vi "Parse Hexadecimal String.vi"(11 "Hex String":string) -> (3 "Bit Stream":bool[](array[boolean]))   [LabVIEW 2019, in "Day 16.lvlib"]
uses:
  Day 16.lvlib
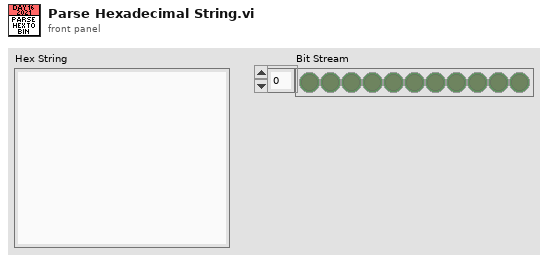
[diagram p1: front panel]
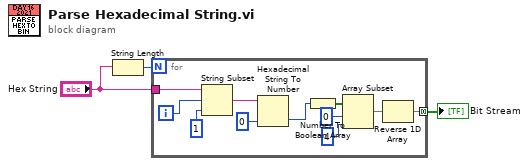
[diagram p0: block diagram]
diagram:
  n1 = String Length(string="Hex String") -> (length=w1:i32)
  n2 = for {
    N: w1 -> [_]
    tunnel: "Hex String" -> [w14]
    tunnel: [w4] -> w3 mode=concatenating
    i -> [w12]
    n3 = String Subset(string=w14, offset (0)=w12, length (rest)=1 ("length (rest)")) -> (substring=w11:string)
    n4 = Hexadecimal String To Number(string=w11, default (0uL)=u8 0 ("default (0 U32)")) -> (number=w10:u8)  [unwired: 1 in, 1 out]
    n5 = Number To Boolean Array(number=w10) -> (Boolean array=w8:bool[])
    n6 = Array Subset(array=w8, index=0, length=4) -> (w5:bool[])
    n7 = Reverse 1D Array(array=w5) -> (reversed array=w4:bool[])
  }
  "Bit Stream" <- w3
